vi "GEOM_ParseROIcmd.vi"(8 "error in":errorcluster, 9 "current rois":T1[](array[typedef]), 10 "cmd":string) -> (0 "error out":errorcluster, 1 "changed":bool, 2 "req rois":T1[](array[typedef]))   [LabVIEW 2016]
uses:
  GEOM_Coords.ctl
  GEOM_Gbls.vi
panel:
  in  "ROIcoords":T1={"xstart"=1, "ystart"=1, "xsize"=1, "ysize"=1}
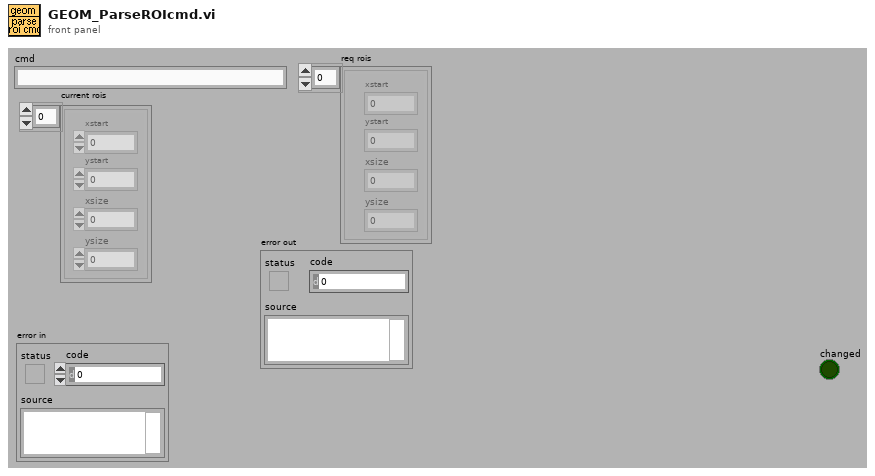
[diagram p1: front panel]
types:
  T1 = typedef "GEOM_Coords.ctl" = cluster{"xstart":u32, "ystart":u32, "xsize":u32, "ysize":u32}
  T2 = cluster{"xstart":bool, "ystart":bool, "xsize":bool, "ysize":bool}
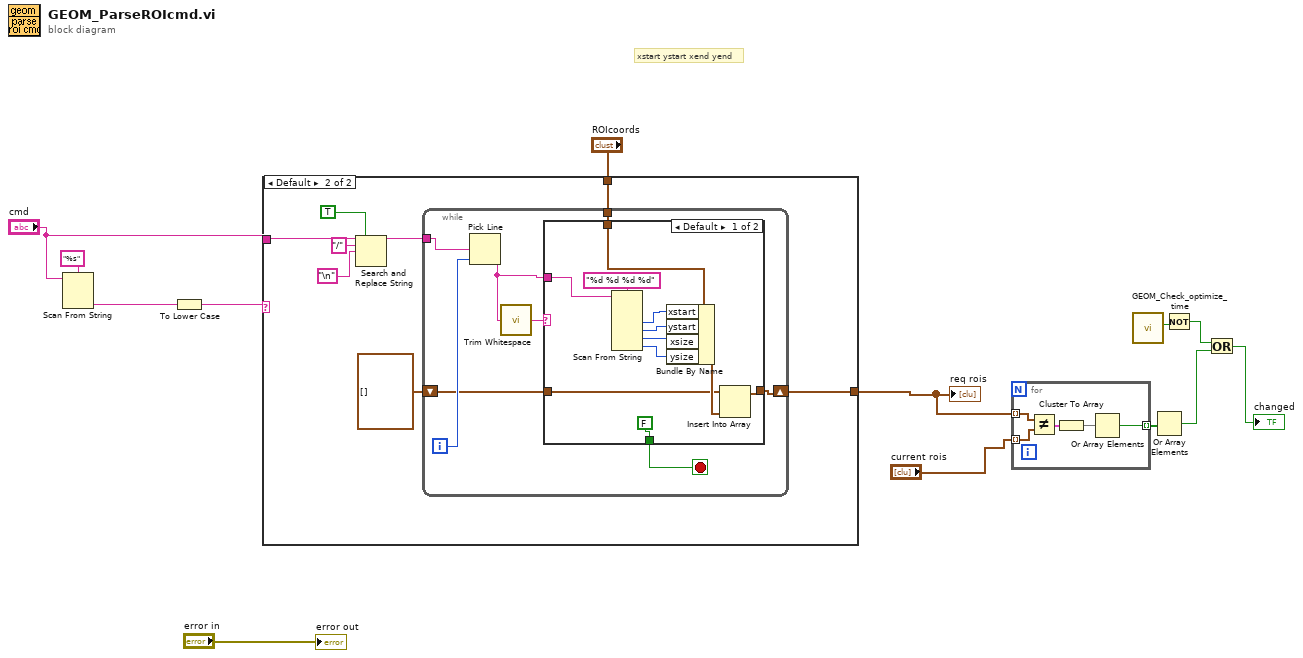
[diagram p0: block diagram]
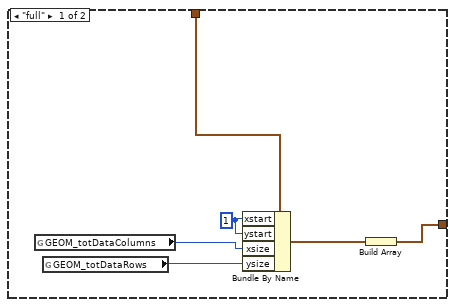
[diagram p2: hidden frame]
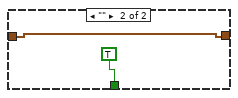
[diagram p3: hidden frame]
diagram:
  # "xstart ystart xend yend"
  n1 = Scan From String(format string="%s", input string="cmd") -> (output 1=w12:string)  [unwired: 2 in, 4 out]
  n2 = To Lower Case(string=w12) -> (all lower case string=w8:string)
  n3 = case shown="Default" w8 {
    tunnel: "cmd" -> [_ w27]
    tunnel: "ROIcoords" -> [w19 w22]
    tunnel: [w17 w21] -> w6
    frame "full" {
      w16 = u32 1 ("xstart")
      n4 = global read "GEOM_Gbls.vi" "GEOM_totDataColumns"() -> (w15:u16)
      n5 = global read "GEOM_Gbls.vi" "GEOM_totDataRows"() -> (w14:u16)
      n6 = Bundle By Name(cluster=w19, "xstart"=w16, "ystart"=w16, "xsize"=w15, "ysize"=w14) -> (w18:T1)
      n7 = Build Array(w18) -> (w17:T1[])
    }
    frame Default {
      n8 = Search and Replace String(replace all?=TRUE ("replace all? (F)"), input string=w27, search string="/", replace string="\n") -> (result string=w23:string)  [unwired: 1 in, 6 out]
      n9 = while {
        tunnel: w23 -> [w34]
        shift-right: [w30] -> w21
        shift-left: T1[] [] -> [w29]
        tunnel: w22 -> [w28]
        i -> [w35]
        stop <- w32 stop-if-true
        n10 = Pick Line(multi-line string=w34, line index=w35) -> (output string=w31:string)  [unwired: 1 out]
        n11 = call <vilib>:"Trim Whitespace.vi"("string"=w31) -> ("trimmed string"=w33:string)  [unwired: 1 in]
        n12 = case shown="Default" w33 {
          tunnel: [FALSE TRUE] -> w32
          tunnel: w31 -> [w45 _]
          tunnel: [w38 w47] -> w30
          tunnel: w29 -> [w37 w47]
          tunnel: w28 -> [w36 _]
          frame Default {
            n13 = Scan From String(format string="%d %d %d %d", input string=w45) -> (output 1=w43:i32, output 2=w42:i32, output 3=w41:i32, output 4=w40:i32)  [unwired: 2 in, 7 out]
            n14 = Bundle By Name(cluster=w36, "xstart"=w43, "ystart"=w42, "xsize"=w41, "ysize"=w40) -> (w39:T1)
            n15 = Insert Into Array(array=w37, new element=w39) -> (w38:T1[])  [unwired: 1 in]
          }
          frame "" {
          }
        }
      }
    }
  }
  "req rois" <- w6
  n16 = for {
    tunnel: w6 -> [w53] mode=indexing
    tunnel: "current rois" -> [w52] mode=indexing
    tunnel: [w49] -> w7 mode=indexing
    n17 = Not Equal?(x=w53, y=w52) -> (x != y?=w51:T2)
    n18 = Cluster To Array(cluster=w51) -> (array=w50:bool[])
    n19 = Or Array Elements(Boolean array=w50) -> (logical OR=w49:bool)
  }
  n20 = call "GEOM_Check_optimize_time.vi"() -> ("optimize"=w4:bool)  [unwired: 11 out]
  n21 = Or Array Elements(Boolean array=w7) -> (logical OR=w2:bool)
  n22 = Not(x=w4) -> (.not. x?=w3:bool)
  n23 = Or(x=w3, y=w2) -> (x .or. y?=→"changed":bool)
  "error out" <- "error in"
